vi "Register NotifyIcon Callback.vi"(0 "NotifyIcon in":refnum<class "NotifyIcon.lvclass">, 11 "error in (no error)":errorcluster) -> (4 "NotifyIcon out":refnum<class "NotifyIcon.lvclass">, 15 "error out":errorcluster)   [LabVIEW 2016, in "NotifyIcon.lvclass"]
doc: "This VI registers the Click, DoubleClick, BalloonTip Open, BalloonTip Close and BalloonTip Click events for the Tray Icon associated with the Notification Icon.\n\nAny previous callback VI registrations are disposed prior to registration.\n\n\nStinus Olsen\nCIM Industrial Systems A/S\n22. Feb. 2011 15:05\nmailto: seo@cim.as"
uses:
  NotifyIcon.lvclass
  NotifyIcon.lvclass/NotifyIcon.ctl
  System.Windows.Forms
panel:
  # "This VI belongs to the NotifyIcon Toolset. \nA toolset that makes it easy to create, control and manipulate a notification icon in the notification area of the Windows taskbar.\nThe toolset requires Microsoft .NET framework 2.0\n\n\nNOTICE -- YOU MUST LEAVE THIS NOTICE IN PLACE.  PER THE TERMS OF THE LICENSE BELOW, YOU MAY SUBLICENSE THIS SOFTWARE \nIN ANY WAY THAT DOES NOT CONFLICT WITH THIS LICENSE.\n\n### BSD License (http://www.opensource.org/licenses/bsd-license.php) Begin ###\n \nCopyright (c) 2011, Stinus Olsen <seo@cim.as>\n\nAll rights reserved.\n\nRedistribution and use in source and binary forms, with or without modification, are permitted provided that the following conditions are met:\n\n    * Redistributions of source code must retain the above copyright notice, this list of conditions and the following disclaimer.\n    * Redistributions in binary form must reproduce the above copyright notice, this list of conditions and the following disclaimer in the \n       documentation and/or other materials provided with the distribution.\n    * Neither the name of CIM Industrial Systems nor the names of its contributors may be used to endorse or promote products derived \n       from this software without specific prior written permission.\n\nTHIS SOFTWARE IS PROVIDED BY THE COPYRIGHT HOLDERS AND CONTRIBUTORS \"AS IS\" AND ANY EXPRESS OR IMPLIED WARRANTIES, \nINCLUDING, BUT NOT LIMITED TO, THE IMPLIED WARRANTIES OF MERCHANTABILITY AND FITNESS FOR A PARTICULAR PURPOSE ARE \nDISCLAIMED. IN NO EVENT SHALL THE COPYRIGHT OWNER OR CONTRIBUTORS BE LIABLE FOR ANY DIRECT, INDIRECT, INCIDENTAL,\n SPECIAL, EXEMPLARY, OR CONSEQUENTIAL DAMAGES (INCLUDING, BUT NOT LIMITED TO, PROCUREMENT OF SUBSTITUTE GOODS OR \nSERVICES; LOSS OF USE, DATA, OR PROFITS; OR BUSINESS INTERRUPTION) HOWEVER CAUSED AND ON ANY THEORY OF LIABILITY, \nWHETHER IN CONTRACT, STRICT LIABILITY, OR TORT (INCLUDING NEGLIGENCE OR OTHERWISE) ARISING IN ANY WAY OUT OF THE USE \nOF THIS SOFTWARE, EVEN IF ADVISED OF THE POSSIBILITY OF SUCH DAMAGE.\n\n### BSD License End ###"
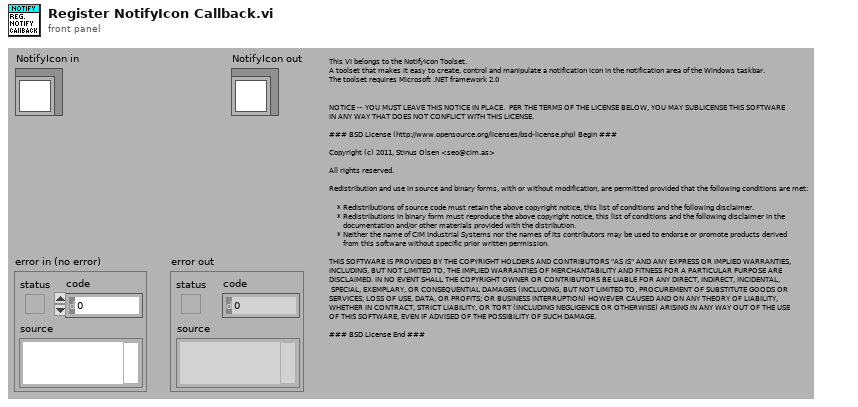
[diagram p1: front panel]
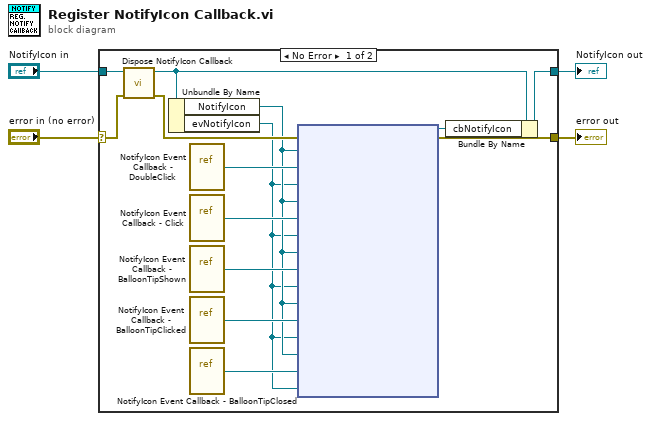
[diagram p0: block diagram]
diagram:
  n1 = case shown="No Error" "error in (no error)" {
    selector: "error in (no error)" -> [w17 w20]
    tunnel: [w11 w20] -> w3
    tunnel: [w12 w19] -> w1
    tunnel: "NotifyIcon in" -> [w18 w19]
    frame No Error {
      n2 = call "Dispose NotifyIcon Callback.vi"("error in (no error)"=w17, "NotifyIcon in"=w18) -> ("error out"=w16:errorcluster, "NotifyIcon out"=w13:refnum<class "NotifyIcon.lvclass">)  [unwired: 8 out]
      n3 = Unbundle By Name(w13) -> ("NotifyIcon"=w7:refnum<k24>, "evNotifyIcon"=w5:refnum<user-event>)
      n4 = vi-ref "NotifyIcon Event Callback - DoubleClick.vi"() -> ("vi reference"=w15:refnum<vi>)
      n5 = vi-ref "NotifyIcon Event Callback - Click.vi"() -> ("vi reference"=w10:refnum<vi>)
      n6 = vi-ref "NotifyIcon Event Callback - BalloonTipShown.vi"() -> ("vi reference"=w9:refnum<vi>)
      n7 = vi-ref "NotifyIcon Event Callback - BalloonTipClicked.vi"() -> ("vi reference"=w8:refnum<vi>)
      n8 = vi-ref "NotifyIcon Event Callback - BalloonTipClosed.vi"() -> ("vi reference"=w6:refnum<vi>)
      n9 = node(w16, w7, w15, w5, w7, w10, w5, w7, w9, w5, w7, w8, w5, w7, w6, w5) -> (w14:refnum<k27>, w11:errorcluster)  [unwired: 1 in]
      n10 = Bundle By Name(cluster=w13, "cbNotifyIcon"=w14) -> (w12:refnum<class "NotifyIcon.lvclass">)
    }
    frame Error {
    }
  }
  "error out" <- w3
  "NotifyIcon out" <- w1
